vi "util.DelimitedStringToArray.vi"(7 "delimiter (,)":string=",", 10 "delimitaed string":string) -> (2 "array out":string[](array[string]))   [LabVIEW 2024]
panel:
  # "util.DelimitedStringFromArray.vi"
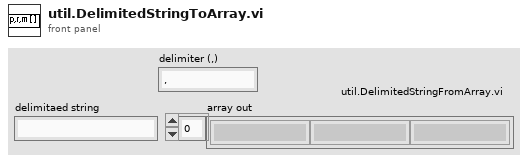
[diagram p1: front panel]
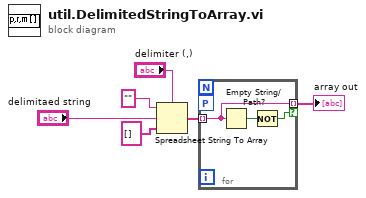
[diagram p0: block diagram]
diagram:
  n1 = Spreadsheet String To Array(delimiter (Tab)="delimiter (,)", format string="", spreadsheet string="delimitaed string", array type (2D Dbl)=string[] []) -> (array=w6:string[])
  n2 = for {
    tunnel: w6 -> [w9] mode=indexing
    tunnel: [w9] -> w1 mode=indexing if=w7
    workers-P: _ -> [_]
    n3 = Empty String/Path?(string/path=w9) -> (empty?=w8:bool)
    n4 = Not(x=w8) -> (.not. x?=w7:bool)
  }
  "array out" <- w1
